vi "METIS_TestIOC.vi"() -> ()   [LabVIEW 2020]
uses:
  d90a4b55-09ae-4f43-bfa2-9b8c1f2ced4f.vi
  <userlib>/caLab/Private/Put_I32-1D_PV-1D.vi
  <userlib>/caLab/Private/Get_PV.vi
panel:
  in  "OK Button":bool
  in  "send":bool
  in  "show":bool=TRUE
  in  "stop":bool
  in  "std":i32=5
  in  "amplitude":dbl=20.0
  in  "ypos":dbl
  out "Intensity Graph":dbl[][](graph)=[[0.3131966385408156, -0.3719194054824131, 0.23345267510587997, 0.501414526387632, 0.9915618098517891, 0.7951711435183322, 0.7770520692901957, 0.9572885462763165, 0.4266860202371128, 0.2602824514012987], [0.5971139193962345, 0.8282797346459745, 1.297812613743599, 1.9501580368662497, 2.8864045590133576, 2.961000657990118, 2.298374943444298, 1.9385955486527697, 1.254315341771823, 0.04258357667043744], [0.6323168707083027, 0.4488178515403488, 2.2459211093616283, 4.05790131844163, 5.742197763142526, 6.80936139569075, 5.260303153014695, 4.022781266980937, 2.5387022125632193, 0.42541594958502793], [0.7548707471220131, 1.6818898427866502, 4.278964212473888, 7.494165542770539, 11.14902238827471, 12.185046051032254, 10.207767961302661, 7.042461192221049, 3.978520358461302, 1.9911109983740998], [1.2187565165963856, 2.6367276481927266, 5.357086117661483, 10.83598637102798, 15.159180269310738, 17.45948905856818, 15.74350240533158, 10.55850051208561, 5.602874968014371, 2.822019015719554], [1.1095052473487188, 2.9799215649337545, 6.933636300818842, 12.211588789250372, 17.45131354805824, 20.15622262568264, 17.744865101682308, 12.203871219623784, 6.26105533426909, 2.400309447093104], [0.6302005306182816, 2.202912915978527, 5.668364349869298, 11.145528829303744, 15.99171534366113, 17.478625699667795, 15.591884275234527, 10.747124157499012, 5.5833771508940435, 2.6610054081022474], [0.3232940748915436, 1.5319577946196734, 3.987670408135723, 7.7753539841303425, 11.035680145982068, 11.954579792806442, 11.04109255650931, 7.753929713227908, 3.5519515316259618, 2.0287201176452796], [0.5564380067991861, 0.4856533963890798, 2.549587054356384, 4.19616574100443, 5.685485157137135, 6.755730038087956, 5.3340316071756115, 4.196898690561765, 2.3202163295831832, 0.6334693718682476], [0.17344664017804434, 0.5308393513043421, 1.1625085552018186, 1.2617013802183377, 2.0364396063526002, 3.0189431667498585, 2.8269534185346163, 1.5046979548585098, 0.565356905040169, 0.49021894750975537]]
  in  "Min":i32=10
  in  "Bin":i32=5
  in  "X":i32=10
  out "PV Errors":errorcluster[](array[cluster])=[{"status"=FALSE, "code"=7192, "source"="Virtual circuit disconnect"}]
  out "Status":bool=TRUE
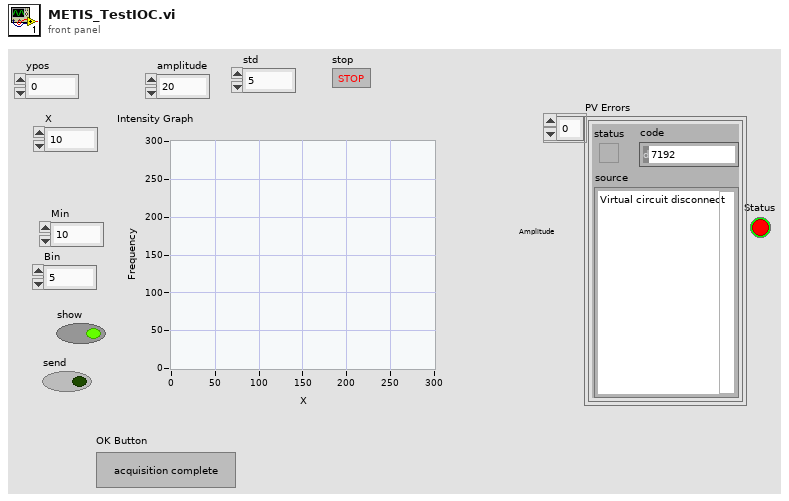
[diagram p1: front panel]
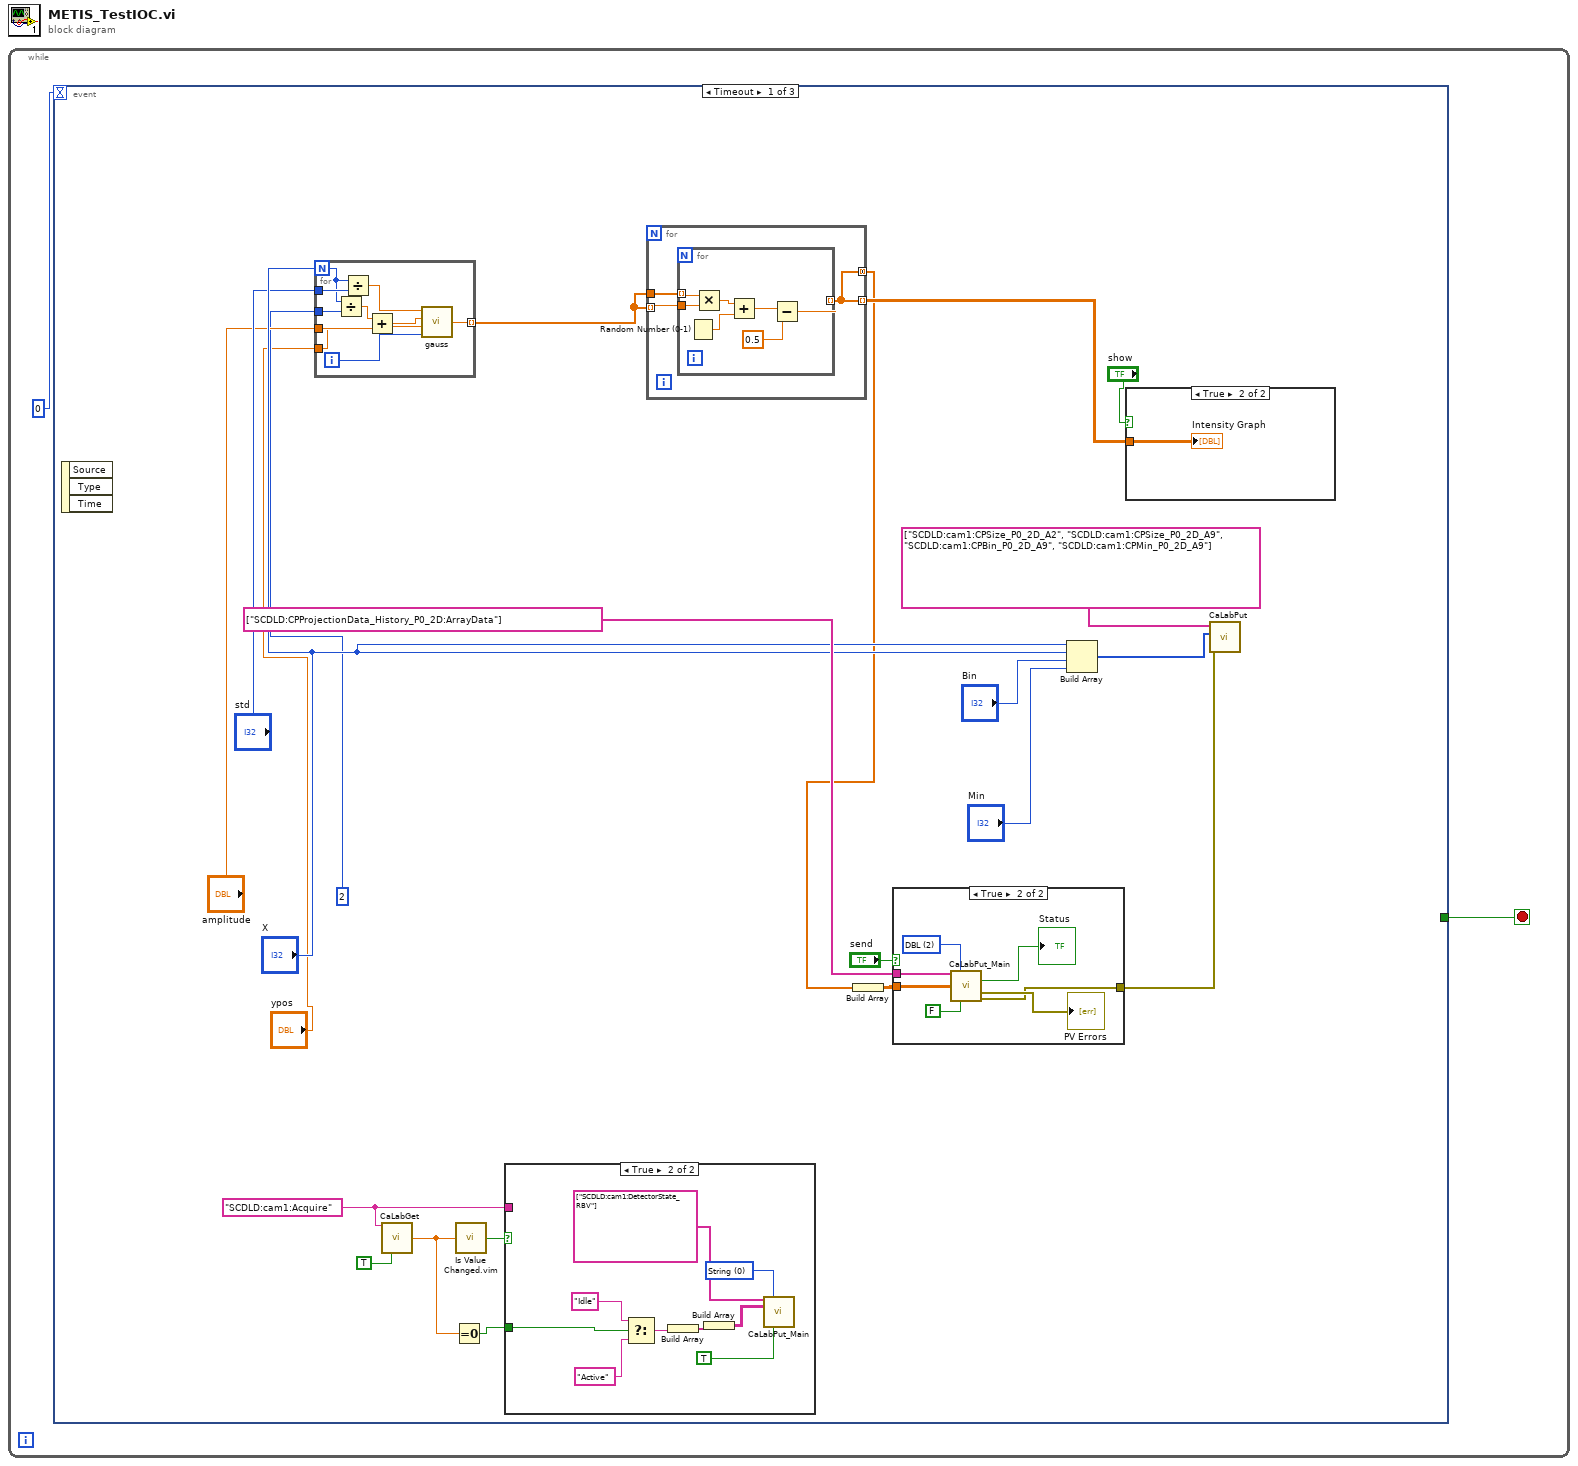
[diagram p0: block diagram]
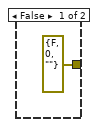
[diagram p3: hidden frame]
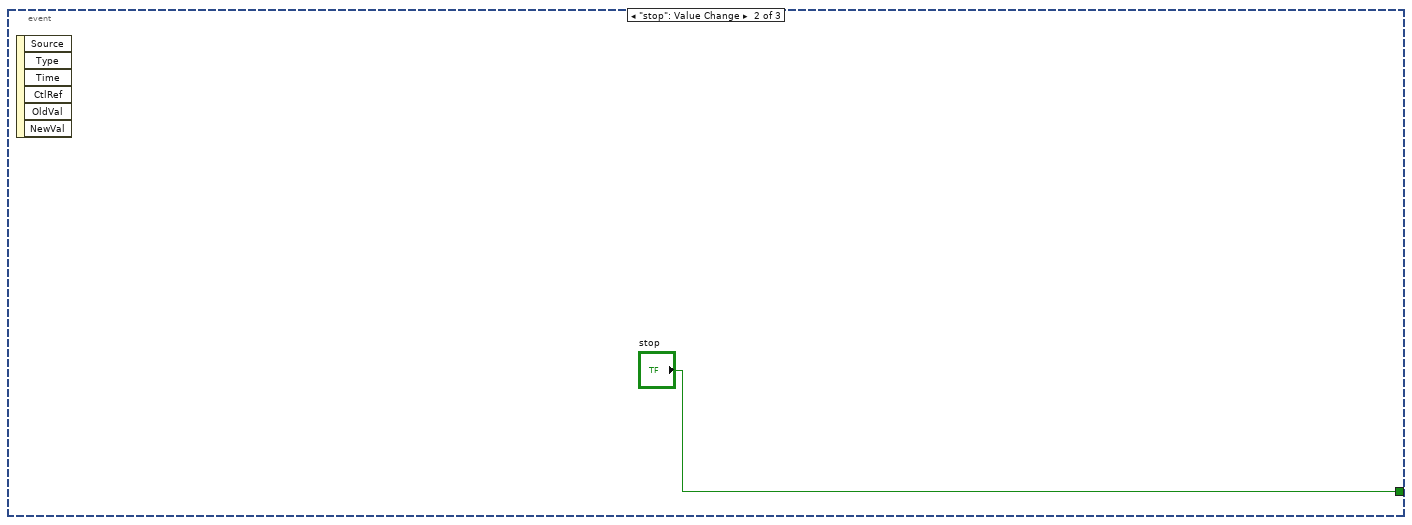
[diagram p5: hidden frame]
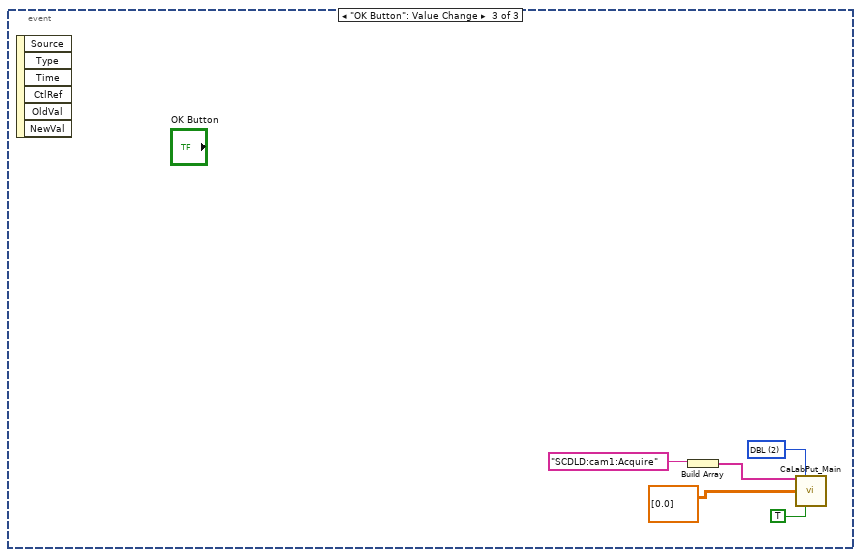
[diagram p6: hidden frame]
diagram:
  n1 = while {
    stop <- w1 stop-if-true
    n2 = event shown="[0] Timeout" {
      selector: _ -> [_ _ _]
      dyn-events: _ -> [_ _ _]
      timeout: 0 -> [_ _ _]
      tunnel: [_ "stop" _] -> w1
      event Timeout {
        w12 = "SCDLD:cam1:Acquire" ("String")
        n3 = event-data() -> ()  [unwired: 1 in, 3 out]
        n4 = for {
          N: "X" -> [w40]
          tunnel: "std" -> [w44]
          tunnel: "amplitude" -> [w41]
          tunnel: 2 ("y") -> [w39]
          tunnel: "ypos" -> [w37]
          tunnel: [w35] -> w5 mode=indexing
          i -> [w42]
          n5 = Divide(x=w40, y=w39) -> (x/y=w38:dbl)
          n6 = Divide(x=w40, y=w44) -> (x/y=w43:dbl)
          n7 = Add(x=w38, y=w37) -> (x+y=w36:dbl)
          n8 = call "gauss.vi"("X"=w42, "amplitude"=w41, "center"=w36, "std. dev."=w43) -> ("y"=w35:dbl)
        }
        n9 = call-poly <userlib>:"CaLabGet.vi"("PV Name"=w12, "NoMDEL(F)"=TRUE) -> ("1rst Value (number)"=w14:dbl)  [unwired: 7 in, 6 out]
        n10 = Equal To 0?(x=w14) -> (x = 0?=w13:bool)
        n11 = call "Is Value Changed.vim"("value"=w14) -> ("changed or first call?"=w15:bool)
        n12 = case shown="True" w15 {
          tunnel: w13 -> [_ w47]
          tunnel: w12 -> [_ _]
          frame False {
          }
          frame True {
            w46 = 0 items=["String", "SGL", "DBL", "I8", "I16", "I32", "I64"] ("Data Type")
            n13 = Select(t="Idle" ("String"), s=w47, f="Active" ("String")) -> (s? t:f=w50:string)
            n14 = Build Array(w50) -> (w49:string[])
            n15 = Build Array(w49) -> (w48:string[][])
            n16 = call <userlib>:"CaLabPut_Main.vi"("PV Names"=string[] ["SCDLD:cam1:DetectorState_RBV"], "Data Type"=w46, "Values [String]"=w48, "Synchronous"=TRUE) -> ()  [unwired: 8 in, 4 out]
          }
        }
        n17 = for {
          tunnel: w5 -> [w26] mode=indexing
          tunnel: w5 -> [w27]
          tunnel: [w25] -> w4 mode=indexing
          tunnel: [w25] -> w3 mode=concatenating
          n18 = for {
            tunnel: w27 -> [w34] mode=indexing
            tunnel: w26 -> [w33]
            tunnel: [w28] -> w25 mode=indexing
            n19 = Random Number (0-1)() -> (number: 0 to 1=w29:dbl)
            n20 = Multiply(x=w34, y=w33) -> (x*y=w30:dbl)
            n21 = Add(x=w30, y=w29) -> (x+y=w32:dbl)
            n22 = Subtract(x=w32, y=0.5) -> (x-y=w28:dbl)
          }
        }
        n23 = Build Array(w3) -> (w24:dbl[][])
        n24 = case shown="True" "send" {
          tunnel: w24 -> [_ w61]
          tunnel: [errorcluster {"status"=FALSE, "code"=0, "source"=""} ("Error out") w58] -> w20
          tunnel: string[] ["SCDLD:CPProjectionData_History_P0_2D:ArrayData"] -> [_ w57]
          frame False {
          }
          frame True {
            w56 = 2 items=["String", "SGL", "DBL", "I8", "I16", "I32", "I64"] ("Data Type")
            n25 = call <userlib>:"CaLabPut_Main.vi"("PV Names"=w57, "Data Type"=w56, "Values [DBL]"=w61, "Synchronous"=FALSE) -> ("Status"=→"Status":bool, "PV Errors"=→"PV Errors":errorcluster[], "Error out"=w58:errorcluster)  [unwired: 8 in, 1 out]
          }
        }
        n26 = Build Array("X", "X", "Bin", "Min") -> (w21:i32[])
        n27 = case shown="True" "show" {
          tunnel: w4 -> [_ w62]
          frame False {
          }
          frame True {
            "Intensity Graph" <- w62
          }
        }
        n28 = call-poly <userlib>:"CaLabPut.vi"("Error in (no error)"=w20, "Values"=w21, "PV Names"=string[] ["SCDLD:cam1:CPSize_P0_2D_A2", "SCDLD:cam1:CPSize_P0_2D_A9", "SCDLD:cam1:CPBin_P0_2D_A9", "SCDLD:cam1:CPMin_P0_2D_A9"]) -> ()  [unwired: 5 in, 4 out]
      }
      event "stop": Value Change {
        n29 = event-data() -> ()  [unwired: 1 in, 6 out]
      }
      event "OK Button": Value Change {
        w68 = 2 items=["String", "SGL", "DBL", "I8", "I16", "I32", "I64"] ("Data Type")
        n30 = event-data() -> ()  [unwired: 1 in, 6 out]
        n31 = Build Array("SCDLD:cam1:Acquire" ("String")) -> (w65:string[])
        n32 = call <userlib>:"CaLabPut_Main.vi"("PV Names"=w65, "Data Type"=w68, "Values [DBL]"=dbl[][] [[0.0]], "Synchronous"=TRUE) -> ()  [unwired: 8 in, 4 out]
      }
    }
  }
